vi "小三轮的 Join HDC Bank3 DIO.vi"(1 "IN 7:6":fxp<+,2,2>, 2 "IN 5:4":fxp<+,2,2>, 3 "IN 3:2":fxp<+,2,2>, 4 "IN 1:0":fxp<+,2,2>) -> (0 "OUT 7:0":u8)   [LabVIEW 2017]
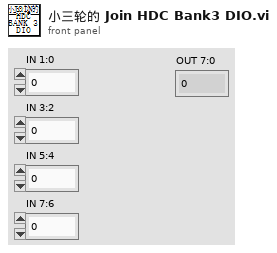
[diagram p1: front panel]
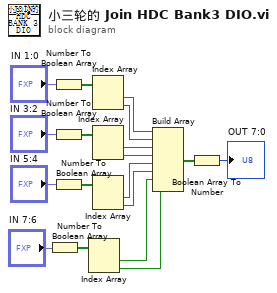
[diagram p0: block diagram]
diagram:
  n1 = Number To Boolean Array(number="IN 7:6") -> (Boolean array=w4:bool[])
  n2 = Number To Boolean Array(number="IN 1:0") -> (Boolean array=w18:bool[])
  n3 = Number To Boolean Array(number="IN 3:2") -> (Boolean array=w17:bool[])
  n4 = Number To Boolean Array(number="IN 5:4") -> (Boolean array=w16:bool[])
  n5 = Index Array(array=w4) -> (element #1=w2:bool, element #2=w1:bool)  [unwired: 2 in]
  n6 = Index Array(array=w18) -> (element #1=w15:bool, element #2=w14:bool)  [unwired: 2 in]
  n7 = Index Array(array=w17) -> (element #1=w13:bool, element #2=w12:bool)  [unwired: 2 in]
  n8 = Index Array(array=w16) -> (element #1=w11:bool, element #2=w5:bool)  [unwired: 2 in]
  n9 = Build Array(w15, w14, w13, w12, w11, w5, w2, w1) -> (w10:bool[])
  n10 = Boolean Array To Number(Boolean array=w10) -> (number=→"OUT 7:0":u8)
